vi "scripting_v3.vi"() -> ()   [LabVIEW 2020]
uses:
  <vilib>/numeric/LVNumericRepresentation.ctl
panel:
  out "appended path":path
  out "concatenated string":string
  out "resulting string":string
  out "error out 2":errorcluster
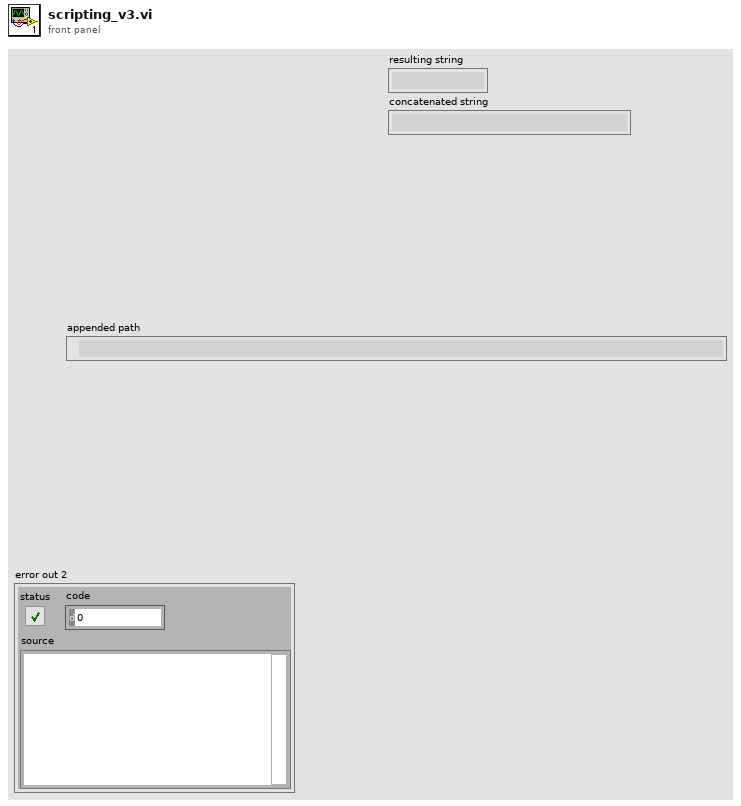
[diagram p1: front panel]
types:
  T1 = typedef "LVNumericRepresentation.ctl" = enum32{"Extended Precision", "Double Precision", "Single Precision", "Long", "Word", "Byte", "Unsigned Long", "Unsigned Word", "Unsigned Byte", "Complex Extended", "Complex Double", "Complex Single", "Quad", "Unsigned Quad", "Fixed-Point"}
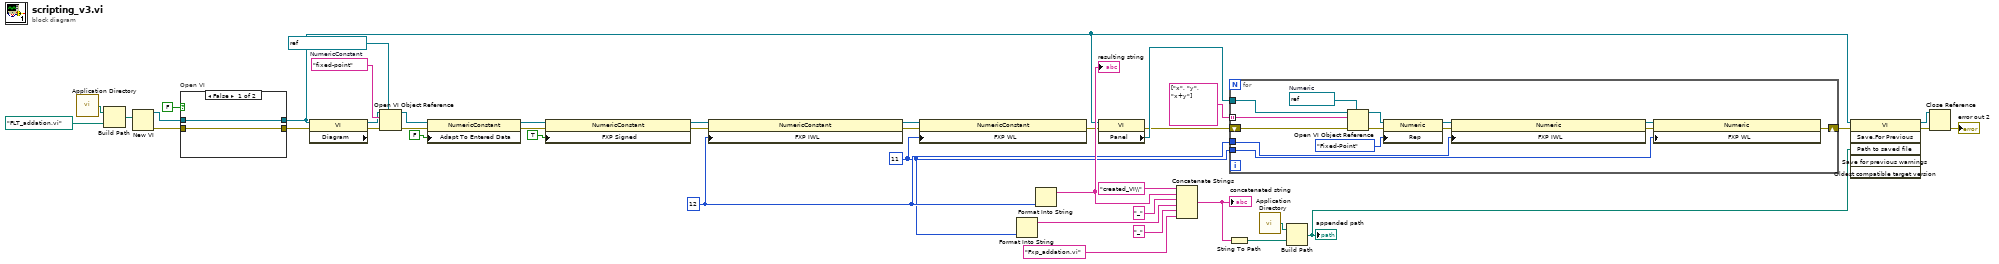
[diagram p0: block diagram]
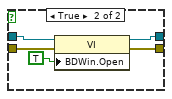
[diagram p2: hidden frame]
diagram:
  w11 = refnum<vi> refnum  # NumericConstant
  w12 = 11 ("Fixed-Point Representation:Bits:Word Length")
  w13 = 12 ("Fixed-Point Representation:Bits:Integer Word Length")
  n1 = call <vilib>:"Application Directory.vi"() -> ("Application Directory"=w33:path)
  n2 = Build Path(base path=w33, name or relative path=path "FLT_addation.vi" ("vi path")) -> (appended path=w31:path)
  n3 = New VI(10:w31) -> (0:w41:errorcluster, 3:w42:refnum<vi>)  [unwired: 6 in]
  n4 = case "Open VI" shown="False" FALSE {
    tunnel: w42 -> [w43 w49]
    tunnel: w41 -> [w44 w48]
    tunnel: [w43 w46] -> w18
    tunnel: [w44 w45] -> w19
    frame False {
    }
    frame True {
      n5 = property class="VI"(reference=w49, error in=w48, "BDWin.Open"=TRUE ("Block Diagram Window:Open")) -> (reference out=w46:refnum<vi>, error out=w45:errorcluster)
    }
  }
  n6 = property on="Property Node" class="VI" props=["Diagram"](reference=w18, error in=w19) -> (reference out=w3:refnum<vi>, error out=w1:errorcluster)  [unwired: 1 out]
  n7 = Open VI Object Reference(7:w11, 8:w1, 10:"fixed-point" ("name/order"), 11:w3) -> (0:w2:errorcluster, 3:w7:refnum<vi>)
  n8 = property on="Property Node" class="NumericConstant"(reference=w7, error in=w2, "Adapt To Entered Data"=FALSE) -> (reference out=w6:refnum<vi>, error out=w5:errorcluster)
  n9 = property on="Property Node" class="NumericConstant"(reference=w6, error in=w5, "FXP Signed"=TRUE ("Fixed-Point Representation:Bits:Signed")) -> (reference out=w10:refnum<vi>, error out=w9:errorcluster)
  n10 = property on="Property Node" class="NumericConstant"(reference=w10, error in=w9, "FXP IWL"=w13) -> (reference out=w16:refnum<vi>, error out=w15:errorcluster)
  n11 = property on="Property Node" class="NumericConstant"(reference=w16, error in=w15, "FXP WL"=w12) -> (error out=w14:errorcluster)  [unwired: 1 out]
  n12 = Format Into String(w12) -> (resulting string=w26:string)  [unwired: 3 in, 1 out]
  n13 = Format Into String(w13) -> (resulting string=w28:string)  [unwired: 3 in, 1 out]
  "resulting string" <- w28
  n14 = property on="Property Node" class="VI"(reference=w18, error in=w14) -> (error out=w35:errorcluster, "Panel"=w36:refnum<vi>)  [unwired: 1 out]
  n15 = Concatenate Strings("created_VI\\" ("string"), w28, "_" ("string"), w26, "_" ("string"), "Fxp_addation.vi" ("string")) -> (w24:string)
  "concatenated string" <- w24
  n16 = String To Path(string=w24) -> (path=w22:path)
  n17 = for {
    tunnel: w36 -> [w61]
    tunnel: w13 -> [w52]
    tunnel: w12 -> [w51]
    shift-right: [w53] -> w34
    shift-left: w35 -> [w59]
    tunnel: string[] ["x", "y", "x+y"] -> [w50] mode=indexing
    w63 = refnum<vi> refnum  # Numeric
    n18 = Open VI Object Reference(7:w63, 8:w59, 10:w50, 11:w61) -> (0:w60:errorcluster, 3:w62:refnum<vi>)
    n19 = property on="Property Node" class="Numeric"(reference=w62, error in=w60, "Rep"=LVNumericRepresentation."Fixed-Point" ("new representation")) -> (reference out=w57:refnum<vi>, error out=w56:errorcluster)
    n20 = property on="Property Node" class="Numeric"(reference=w57, error in=w56, "FXP IWL"=w52) -> (reference out=w55:refnum<vi>, error out=w54:errorcluster)
    n21 = property on="Property Node" class="Numeric"(reference=w55, error in=w54, "FXP WL"=w51) -> (error out=w53:errorcluster)  [unwired: 1 out]
  }
  n22 = call <vilib>:"Application Directory.vi"() -> ("Application Directory"=w30:path)
  n23 = Build Path(base path=w30, name or relative path=w22) -> (appended path=w29:path)
  "appended path" <- w29
  n24 = invoke class="VI" method="Save.For Previous"(reference=w18, error in=w34, "Path to saved file"=w29) -> (reference out=w40:refnum<vi>, error out=w39:errorcluster)  [unwired: 3 in, 4 out]
  n25 = Close Reference(reference=w40, error in (no error)=w39) -> (error out=→"error out 2":errorcluster)
